vi "UDP Data Link - Pages - Rx Channels Section Page.vi"(8 "error in (no error)":errorcluster, 11 "Node Ptr":T1 format="%.0x") -> (0 "error out":errorcluster)   [LabVIEW 2012, in "UDP Data Link System Explorer.lvlib"]
uses:
  UDP Data Link System Explorer.lvlib
  <vilib>/NI Veristand/Custom Device API/Custom Device Item Ref.ctl
  TypeDefs/UDP Data Link - TypeDefs - Rx Channels Section Page References.ctl
  Shared/UDP Data Link Global.vi
  <vilib>/NI Veristand/Custom Device API/Set Item Property (I32 Array).vi
  <vilib>/NI Veristand/Custom Device API/Custom Device API.lvlib
  Shared/UDP Data Link Shared.lvlib
panel:
  in  "Rx Channels":i32[](listbox)
  in  "Header":cluster{"Section Name":string}={"Section Name"="Transmit Settings"}
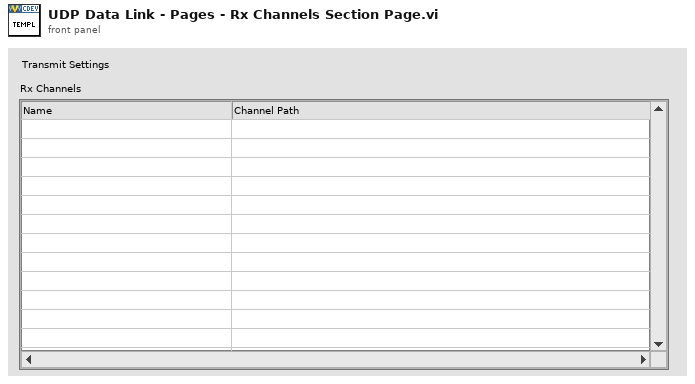
[diagram p1: front panel]
types:
  T1 = typedef "Custom Device API.lvlib/Custom Device Item Ref.ctl" = u64
  T2 = typedef "UDP Data Link System Explorer.lvlib/UDP Data Link - TypeDefs - Rx Channels Section Page References.ctl" = cluster{"Rx Channels":refnum<vi>}
  T3 = typedef "Custom Device API.lvlib/Custom Device Commands.ctl" = enum16{"Default", "Item renamed", "Shutdown", "Dynamic button pressed"}
  T4 = typedef "Custom Device API.lvlib/Custom Device Item Info.ctl" = cluster{"Name":string, "Is Channel":bool, "GUID":string, "Is Waveform":bool}
  T5 = typedef "LVPoint32TypeDef.ctl" = cluster{"Horizontal":i32, "Vertical":i32}
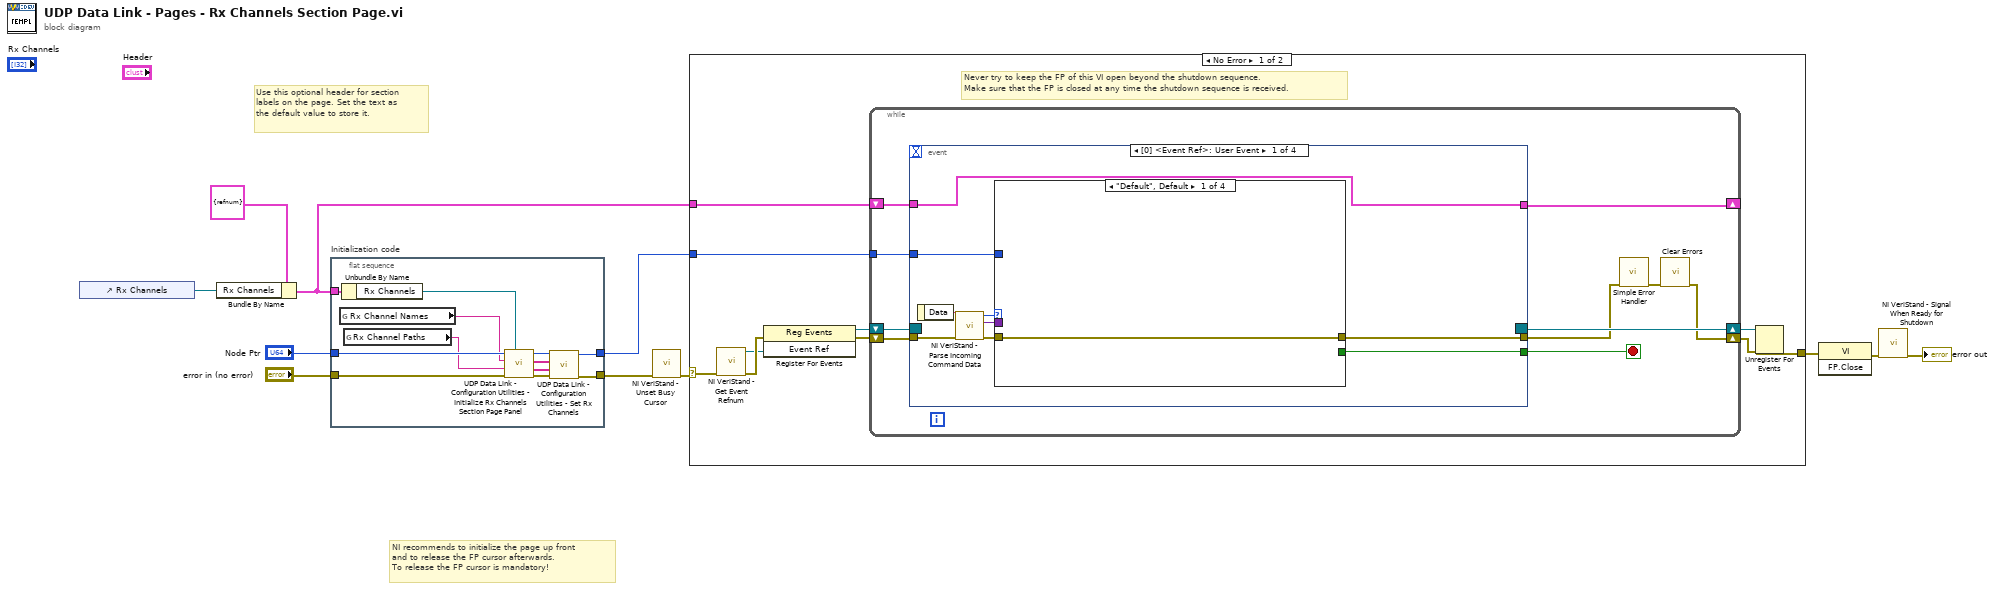
[diagram p0: block diagram]
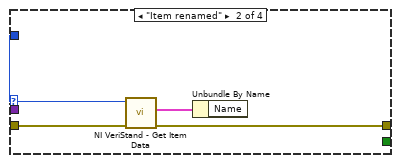
[diagram p2: hidden frame]
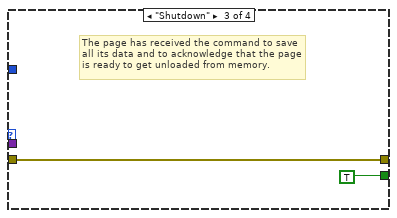
[diagram p3: hidden frame]
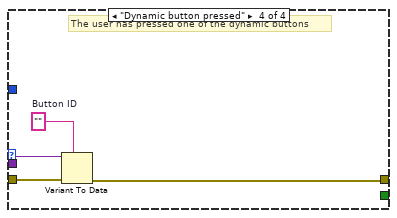
[diagram p4: hidden frame]
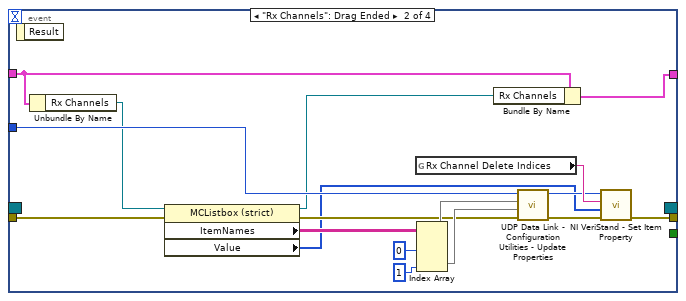
[diagram p5: hidden frame]
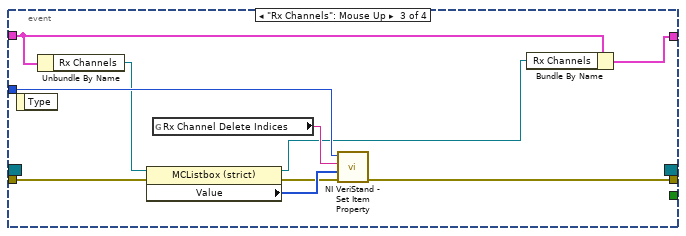
[diagram p6: hidden frame]
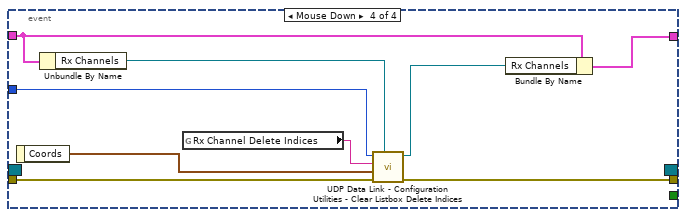
[diagram p7: hidden frame]
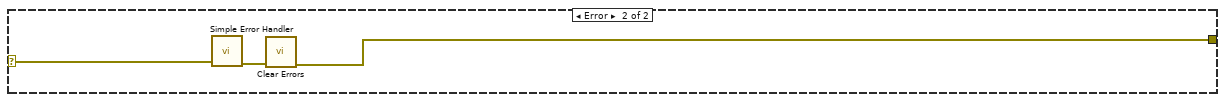
[diagram p8: hidden frame]
diagram:
  # "Use this optional header for section labels on the page. Set the text as the default value to store it."
  # "NI recommends to initialize the page up front\nand to release the FP cursor afterwards.\nTo release the FP cursor is mandatory!"
  n1 = control-ref of="Rx Channels"() -> (w3:refnum<vi>)
  n2 = Bundle By Name(cluster=T2 {"Rx Channels"=refnum} ("Rx Channels Section Cluster"), "Rx Channels"=w3) -> (w2:T2)
  n3 = flat-sequence "Initialization code" {
    tunnel: "error in (no error)" -> [w23]
    tunnel: "Node Ptr" -> [w22]
    tunnel: [w12] -> w7
    tunnel: [w13] -> w4
    tunnel: w2 -> [w21]
    frame #0 {
      n4 = global read "UDP Data Link Global.vi" "Rx Channel Names"() -> (w19:string)
      n5 = Unbundle By Name(w21) -> ("Rx Channels"=w20:refnum<vi>)
      n6 = global read "UDP Data Link Global.vi" "Rx Channel Paths"() -> (w18:string)
      n7 = call "UDP Data Link - Configuration Utilities - Initialize Rx Channels Section Page Panel.vi"("Channels Listbox"=w20, "error in (no error)"=w23, "Channel Paths Property"=w18, "Channel Names Property"=w19, "Item Ref in"=w22) -> ("error out"=w17:errorcluster, "Channel Paths"=w15:string[], "Channel Names"=w16:string[], "Item Ref out"=w14:T1)  [unwired: 3 in]
      n8 = call "UDP Data Link - Configuration Utilities - Set Rx Channels.vi"("error in (no error)"=w17, "Rx Channel Paths"=w15, "Rx Channel Names"=w16, "Item Ref in"=w14) -> ("error out"=w12:errorcluster, "Item Ref out"=w13:T1)  [unwired: 6 in]
    }
  }
  n9 = call <vilib>:"NI VeriStand - Unset Busy Cursor.vi"("error in (no error)"=w7) -> ("error out"=w6:errorcluster)  [unwired: 10 out]
  n10 = case shown="No Error" w6 {
    selector: w6 -> [w25 w102]
    tunnel: [w30 w100] -> w11
    tunnel: w4 -> [w26 _]
    tunnel: w2 -> [w24 _]
    frame No Error {
      # "Never try to keep the FP of this VI open beyond the shutdown sequence.\nMake sure that the FP is closed at any time the shutdown sequence is received."
      n11 = call <vilib>:"NI VeriStand - Get Event Refnum.vi"("error in (no error)"=w25) -> ("error out"=w33:errorcluster, "Event Ref"=w29:refnum<user-event>)  [unwired: 9 out]
      n12 = register-events(error in=w33, w29) -> (reference out=w27:refnum<event-registration>, error out=w28:errorcluster)  [unwired: 1 in]
      n13 = while {
        tunnel: w26 -> [w35]
        shift-right: [w37] -> w31
        shift-left: w28 -> [w42]
        shift-right: [w43] -> w32
        shift-left: w27 -> [w41]
        shift-right: [w34] -> _
        shift-left: w24 -> [w36]
        stop <- w40 stop-if-true
        n14 = event shown="[0] <Event Ref>: User Event" {
          selector: w41 -> [_ _ _ _]
          dyn-events: [_ _ _ _] -> w43
          timeout: _ -> [_ _ _ _]
          tunnel: w42 -> [w52 w71 w84 w98]
          tunnel: [w48 _ _ _] -> w40
          tunnel: [w47 w74 w89 w99] -> w39
          tunnel: w35 -> [w46 w80 w88 w96]
          tunnel: w36 -> [w44 w66 w83 w93]
          tunnel: [w44 w64 w81 w91] -> w34
          event User Event {
            n15 = event-data() -> ("Data"=w51:string)  [unwired: 1 out]
            n16 = call <vilib>:"NI VeriStand - Parse Incoming Command Data.vi"("error in (no error)"=w52, "Incoming data"=w51) -> ("error out"=w50:errorcluster, "Outgoing data"=w45:variant, "Action"=w49:T3)  [unwired: 7 out]
            n17 = case shown="\"Default\", Default" w49 {
              tunnel: w50 -> [w53 w57 w58 w63]
              tunnel: [_ _ TRUE _] -> w48
              tunnel: [w53 w54 w58 w60] -> w47
              tunnel: w46 -> [_ w56 _ _]
              tunnel: w45 -> [_ _ _ w62]
              frame "Default", Default {
              }
              frame "Item renamed" {
                n18 = call <vilib>:"NI VeriStand - Get Item Data.vi"("error in (no error)"=w57, "Item Ref in"=w56) -> ("error out"=w54:errorcluster, "Item Info"=w55:T4)  [unwired: 8 out]
                n19 = Unbundle By Name(w55) -> ()  [unwired: 1 out]
              }
              frame "Shutdown" {
                # "The page has received the command to save all its data and to acknowledge that the page is ready to get unloaded from memory."
              }
              frame "Dynamic button pressed" {
                w61 = ""  # Button ID
                # "The user has pressed one of the dynamic buttons"
                n20 = Variant To Data(error in=w63, type=w61, Variant=w62) -> (error out=w60:errorcluster)  [unwired: 1 out]
              }
            }
          }
          event "Rx Channels": Drag Ended {
            n21 = event-data() -> ()  [unwired: 2 out]
            n22 = Unbundle By Name(w66) -> ("Rx Channels"=w69:refnum<vi>)
            n23 = property class="MCListbox (strict)"(reference=w69, error in=w71) -> (reference out=w65:refnum<vi>, error out=w70:errorcluster, "ItemNames"=w72:string[][], "Value"=w68:i32[])
            n24 = global read "UDP Data Link Global.vi" "Rx Channel Delete Indices"() -> (w75:string)
            n25 = Index Array(array=w72, index (col) #1=0 ("disabled index (col)"), index (col) #2=1 ("index (col)")) -> (element #1=w77:string[], element #2=w76:string[])  [unwired: 2 in]
            n26 = Bundle By Name(cluster=w66, "Rx Channels"=w65) -> (w64:T2)
            n27 = call "UDP Data Link - Configuration Utilities - Update Properties.vi"("error in (no error)"=w70, "Channel Paths"=w76, "Channel Names"=w77, "Item Ref in"=w80) -> ("error out"=w67:errorcluster, "Item Ref out"=w73:T1)  [unwired: 6 in]
            n28 = call-poly <vilib>:"NI VeriStand - Set Item Property.vi"("error in (no error)"=w67, "Value"=w68, "Property Name"=w75, "Item Ref in"=w73) -> ("error out"=w74:errorcluster)  [unwired: 5 in, 2 out]
          }
          event "Rx Channels": Mouse Up {
            n29 = event-data() -> ()  [unwired: 2 out]
            n30 = Unbundle By Name(w83) -> ("Rx Channels"=w87:refnum<vi>)
            n31 = property class="MCListbox (strict)"(reference=w87, error in=w84) -> (reference out=w82:refnum<vi>, error out=w85:errorcluster, "Value"=w86:i32[])
            n32 = global read "UDP Data Link Global.vi" "Rx Channel Delete Indices"() -> (w90:string)
            n33 = call-poly <vilib>:"NI VeriStand - Set Item Property.vi"("error in (no error)"=w85, "Value"=w86, "Property Name"=w90, "Item Ref in"=w88) -> ("error out"=w89:errorcluster)  [unwired: 5 in, 2 out]
            n34 = Bundle By Name(cluster=w83, "Rx Channels"=w82) -> (w81:T2)
          }
          event Mouse Down {
            n35 = event-data() -> ("Coords"=w94:T5)  [unwired: 1 out]
            n36 = Unbundle By Name(w93) -> ("Rx Channels"=w97:refnum<vi>)
            n37 = global read "UDP Data Link Global.vi" "Rx Channel Delete Indices"() -> (w95:string)
            n38 = call "UDP Data Link - Configuration Utilities - Clear Listbox Delete Indices.vi"("Listbox Reference in"=w97, "error in (no error)"=w98, "Pane Coords"=w94, "Delete Property Name"=w95, "Item Ref in"=w96) -> ("error out"=w99:errorcluster, "Listbox Reference out"=w92:refnum<vi>)  [unwired: 5 in]
            n39 = Bundle By Name(cluster=w93, "Rx Channels"=w92) -> (w91:T2)
          }
        }
        n40 = call <vilib>:"Simple Error Handler.vi"("error in (no error)"=w39) -> ("error out"=w38:errorcluster)  [unwired: 1 in, 7 out]
        n41 = call <vilib>:"Clear Errors.vi"("error in (no error)"=w38) -> ("error out"=w37:errorcluster)  [unwired: 6 out]
      }
      n42 = Unregister For Events(event registration refnum=w32, error in=w31) -> (error out=w30:errorcluster)
    }
    frame Error {
      n43 = call <vilib>:"Simple Error Handler.vi"("error in (no error)"=w102) -> ("error out"=w101:errorcluster)  [unwired: 1 in, 7 out]
      n44 = call <vilib>:"Clear Errors.vi"("error in (no error)"=w101) -> ("error out"=w100:errorcluster)  [unwired: 6 out]
    }
  }
  n45 = invoke class="VI" method="FP.Close"(error in=w11) -> (error out=w10:errorcluster)  [unwired: 2 in, 2 out]
  n46 = call <vilib>:"NI VeriStand - Signal When Ready for Shutdown.vi"("error in (no error)"=w10) -> ("error out"=→"error out":errorcluster)  [unwired: 10 out]
